vi "Signal_Generator.vi"() -> ()   [LabVIEW 2018]
uses:
  Global_Signal.vi
  <vilib>/measure/NI_MABase.lvlib
panel:
  in  "?":T1={"Sampling Rate"=1000.0, "Number of samples"=1000.0}
  out "Square_OR_Not":bool
  in  "Square_Wave_Duty_Cycle":dbl=50.0
  out "?":dbl(knob) scale=0.0..10.0
  out "?":dbl(knob) scale=0.0..100.0
  out "?":dbl(knob) scale=0.0..100.0
  out "?":dbl(knob) scale=0.0..10000.0
  in  "Offset":dbl
  in  "Phase":dbl
  out "?":dbl(knob) scale=0.0..100.0
  in  "Pause":bool=TRUE
  out "Running":bool
  in  "Amplitude":dbl=5.0
  in  "Frequence(<10KHz)":dbl=20.0 max=10000.0
  in  "Signal_Type":u16(ring) items=["Sine Wave", "Triangle Wave", "Square Wave", "Sawtooth Wave"]
  out "Waveform Graph":waveform(dbl)(graph)
  in  "Power":bool
  # "Virtual Waveform Generator"
  # "Only For Square Wave Duty Cycle"
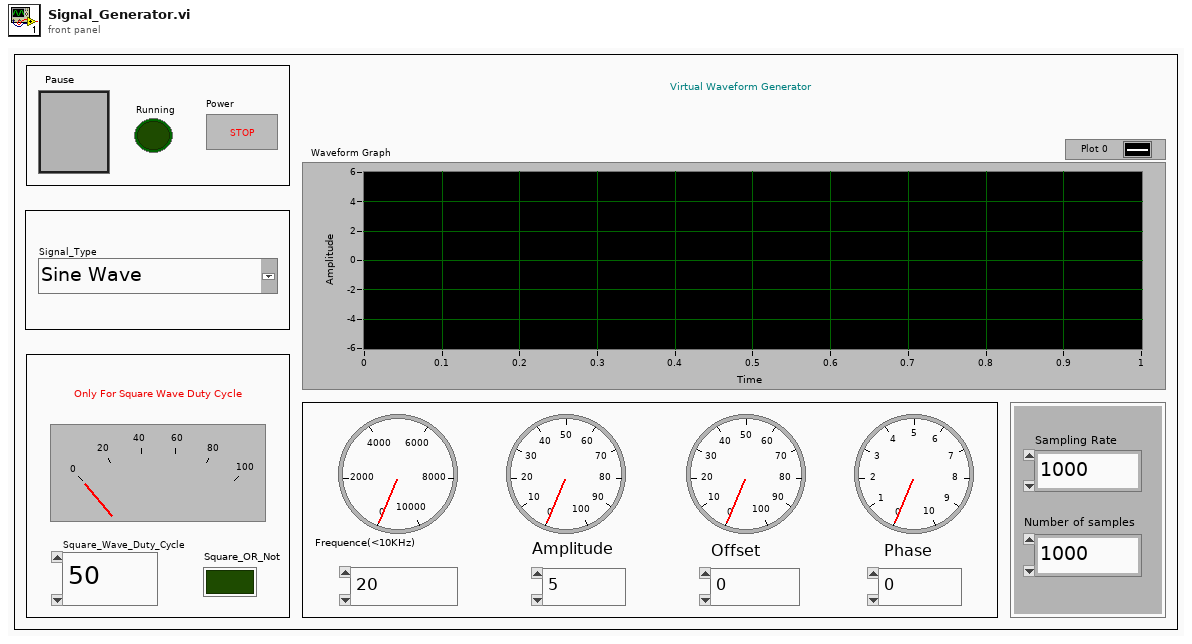
[diagram p1: front panel]
types:
  T1 = cluster{"Sampling Rate":dbl, "Number of samples":dbl}
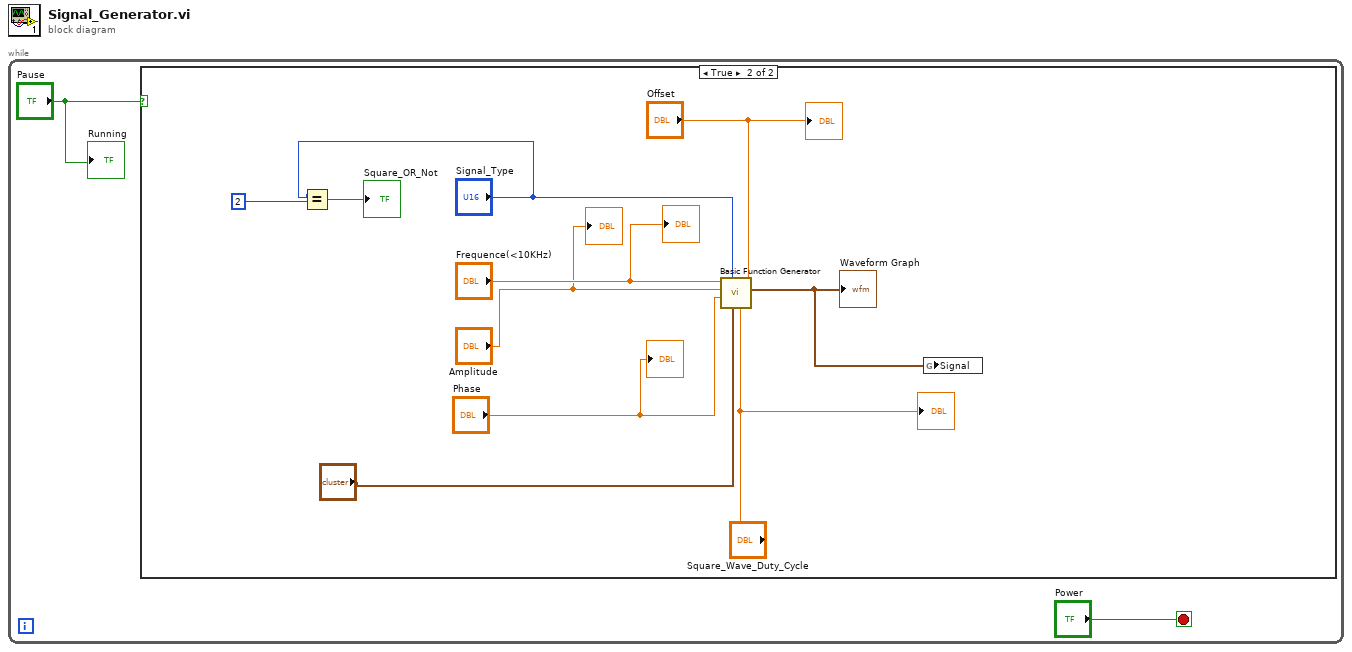
[diagram p0: block diagram]
diagram:
  n1 = while {
    stop <- "Power" stop-if-true
    n2 = case shown="True" "Pause" {
      frame False {
      }
      frame True {
        n3 = Equal?(x="Signal_Type", y=2) -> (x = y?=→"Square_OR_Not":bool)
        n4 = call <vilib>:"Basic Function Generator.vi"("offset"="Offset", "square wave duty cycle (%)"="Square_Wave_Duty_Cycle", "sampling info"="?", "signal type"="Signal_Type", "phase"="Phase", "amplitude"="Amplitude", "frequency"="Frequence(<10KHz)") -> ("signal out"=w3:waveform(dbl))  [unwired: 2 in, 2 out]
        "Waveform Graph" <- w3
        n5 = global write "Global_Signal.vi" "Signal"(w3) -> ()
        "?" <- "Square_Wave_Duty_Cycle"
        "?" <- "Frequence(<10KHz)"
        "?" <- "Amplitude"
        "?" <- "Offset"
        "?" <- "Phase"
      }
    }
    "Running" <- "Pause"
  }
